vi "Get Type.vi"(11 "Assertion in":refnum<class "Assertion.lvclass">) -> (3 "Type":string)   [LabVIEW 2019, in "Assertion.lvclass"]
uses:
  <vilib>/gpm_packages/@cs/data-type-serializer/source/Assertion/Assertion.lvclass
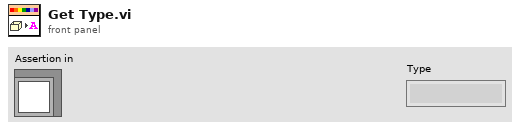
[diagram p1: front panel]
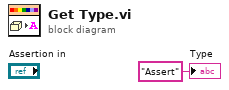
[diagram p0: block diagram]
diagram:
  "Type" <- "Assert" ("Type")
